vi "PC_Pub_imgFile connectRT.vi"(8 "error in (no error)":errorcluster, 10 "IPV4":string="100.100.0.123", 11 "imgFile in":refnum<class "PC_Pub_imgFile.lvclass">=refnum) -> (0 "error out":errorcluster, 3 "imgFile out":refnum<class "PC_Pub_imgFile.lvclass">)   [LabVIEW 2018, in "PC_Pub_imgFile.lvclass"]
uses:
  PC_Pub_imgFile.lvclass
  PC_Pub_imgFile.lvclass/PC_Pub_imgFile.ctl
  <vilib>/nisyscfg/nisyscfg.lvlib
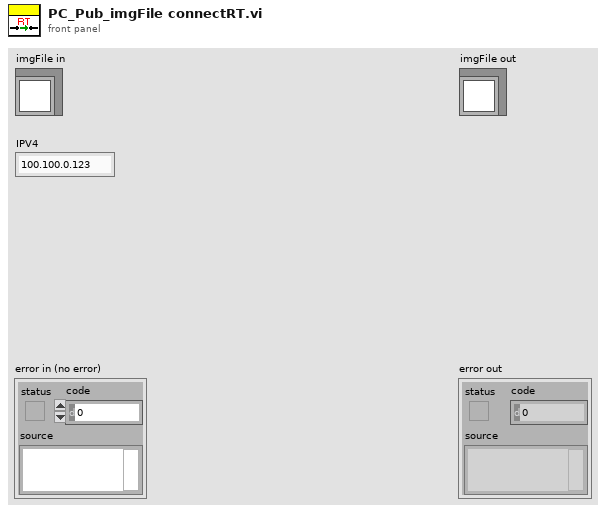
[diagram p1: front panel]
types:
  T1 = enum8{"Enabled", "Disabled", "Disabled and Grayed Out"}
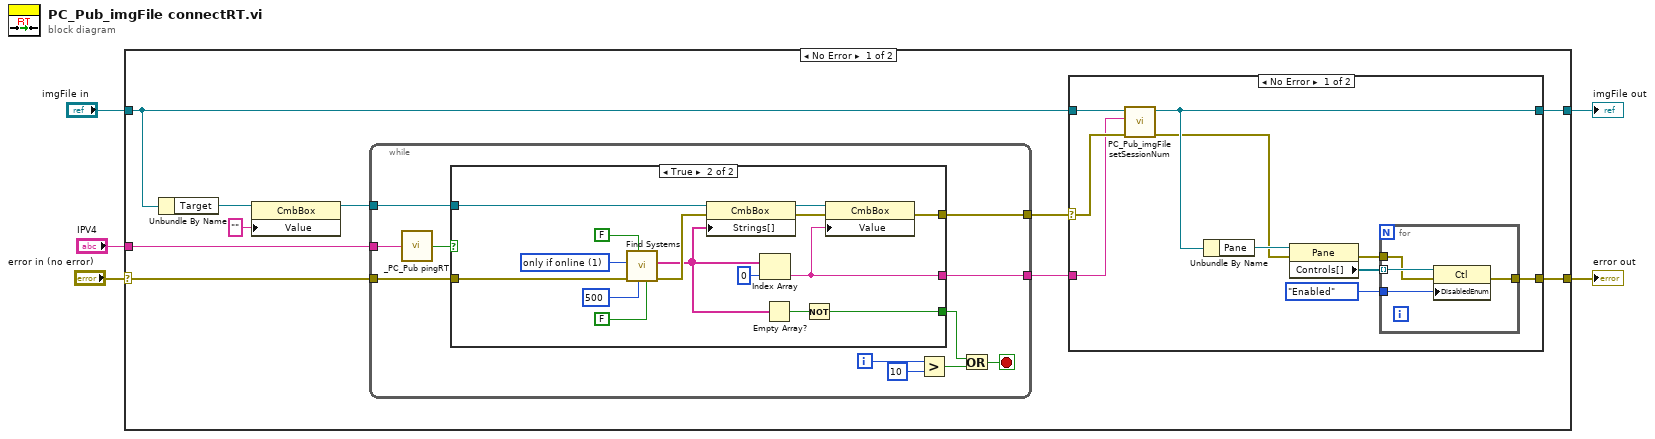
[diagram p0: block diagram]
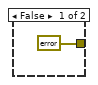
[diagram p2: hidden frame]
diagram:
  n1 = case shown="No Error" "error in (no error)" {
    selector: "error in (no error)" -> [w15 w60]
    tunnel: [w14 w60] -> w4
    tunnel: [w10 w59] -> w2
    tunnel: "imgFile in" -> [w13 w59]
    tunnel: "IPV4" -> [w9 _]
    frame No Error {
      n2 = Unbundle By Name(w13) -> ("Target"=w8:refnum<vi>)
      n3 = property class="CmbBox"(reference=w8, "Value"="") -> (reference out=w7:refnum<vi>)  [unwired: 1 in, 1 out]
      n4 = while {
        tunnel: w7 -> [w25]
        tunnel: [w23] -> w12
        tunnel: w9 -> [w21]
        tunnel: w15 -> [w24]
        tunnel: [w22] -> w11
        i -> [w20]
        stop <- w16 stop-if-true
        n5 = call "_PC_Pub pingRT.vi"("IPV4"=w21) -> ("valid"=w26:bool)  [unwired: 1 in]
        n6 = case shown="True" w26 {
          tunnel: w25 -> [_ w38]
          tunnel: w24 -> [_ w31]
          tunnel: [_ w33] -> w23
          tunnel: [errorcluster {"status"=TRUE, "code"=0, "source"=""} ("error out") w32] -> w22
          tunnel: [_ w28] -> w18
          frame False {
          }
          frame True {
            w39 = u32 1 items=["none"=0, "only if online"=1, "all"=3] ("Include Cached Results (all)")
            n7 = call <vilib>:"Find Systems.vi"("Only Installable Systems (F)"=FALSE, "Timeout (4000 ms)"=u32 500, "Detect Online Systems (T)"=FALSE, "error in (no error)"=w31, "Include Cached Results (all)"=w39) -> ("error out"=w34:errorcluster, "Detected Systems"=w30:string[])  [unwired: 4 in, 1 out]
            n8 = property class="CmbBox"(reference=w38, error in=w34, "Strings[]"=w30) -> (reference out=w37:refnum<vi>, error out=w36:errorcluster)
            n9 = Index Array(array=w30, index=0) -> (element=w33:string)
            n10 = Empty Array?(array=w30) -> (empty?=w29:bool)
            n11 = Not(x=w29) -> (.not. x?=w28:bool)
            n12 = property class="CmbBox"(reference=w37, error in=w36, "Value"=w33) -> (error out=w32:errorcluster)  [unwired: 1 out]
          }
        }
        n13 = Greater?(x=w20, y=10) -> (0:w17:bool)
        n14 = Or(x=w18, y=w17) -> (x .or. y?=w16:bool)
      }
      n15 = case shown="No Error" w11 {
        selector: w11 -> [w45 w58]
        tunnel: [w49 w58] -> w14
        tunnel: w13 -> [w47 w57]
        tunnel: w12 -> [w44 _]
        tunnel: [w46 w57] -> w10
        frame No Error {
          n16 = call "PC_Pub_imgFile setSessionNum.vi"("error in (no error)"=w45, "newSessionString"=w44, "imgFile in"=w47) -> ("error out"=w43:errorcluster, "imgFile out"=w46:refnum<class "PC_Pub_imgFile.lvclass">)  [unwired: 7 in]
          n17 = Unbundle By Name(w46) -> ("Pane"=w48:refnum<vi>)
          n18 = property class="Pane"(reference=w48, error in=w43) -> (error out=w50:errorcluster, "Controls[]"=w52:refnum<vi>[])  [unwired: 1 out]
          n19 = for {
            tunnel: w52 -> [w54] mode=indexing
            tunnel: T1."Enabled" ("Disabled") -> [w55]
            tunnel: w50 -> [w53]
            tunnel: [w56] -> w49
            n20 = property class="Ctl"(reference=w54, error in=w53, "DisabledEnum"=w55) -> (error out=w56:errorcluster)  [unwired: 1 out]
          }
        }
        frame Error {
        }
      }
    }
    frame Error {
    }
  }
  "error out" <- w4
  "imgFile out" <- w2
